vi "Create Find and Replace Array for Word.vi"(7 "Language":string, 8 "error in":errorcluster, 10 "Mathcad Output":T1, 11 "DesignRequest":T2) -> (0 "error out":errorcluster, 3 "Find-Replace":cluster{"Find":string, "Replace":string}[](array[cluster]))   [LabVIEW 2012, in "Design Server.lvlib"]
uses:
  Design Server.lvlib
  Design Request.ctl
  Variable cluster.ctl
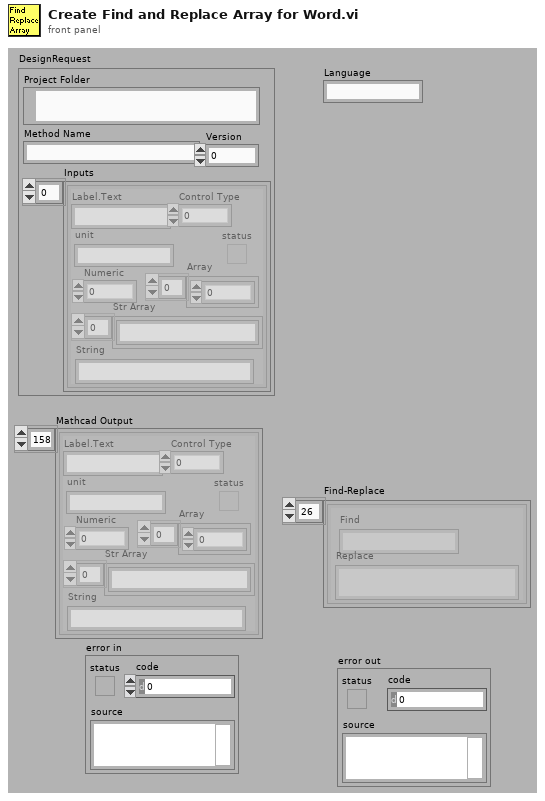
[diagram p1: front panel]
types:
  T1 = typedef "Design Server.lvlib/Variable cluster.ctl" = cluster{"Label.Text":string, "Control Type":u32, "Numeric":dbl, "Array":dbl[], "status":bool, "Str Array":string[], "String":string, "unit":string}[]
  T2 = typedef "Design Server.lvlib/Design Request.ctl" = cluster{"Project Folder":path, "Method Name":string, "Inputs":T1, "Version":i32}
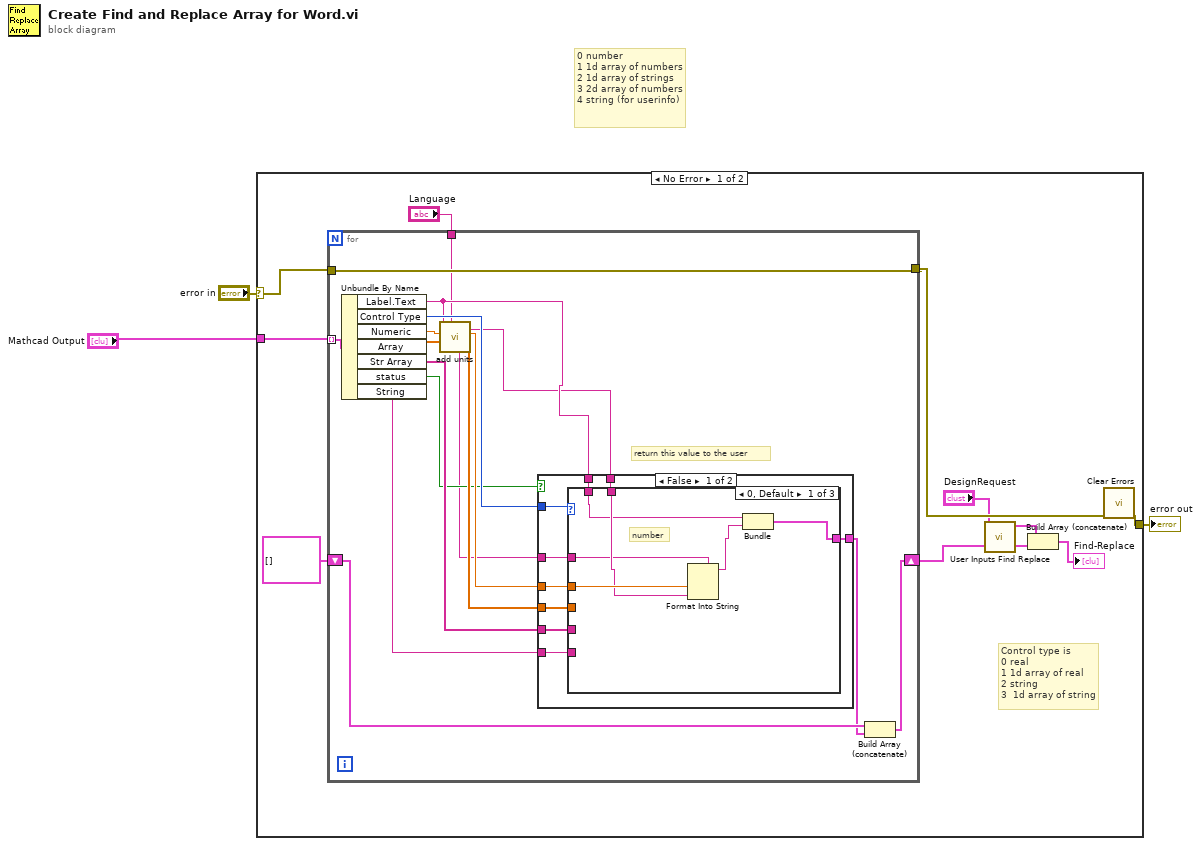
[diagram p0: block diagram]
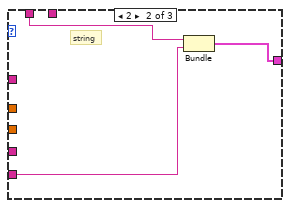
[diagram p2: hidden frame]
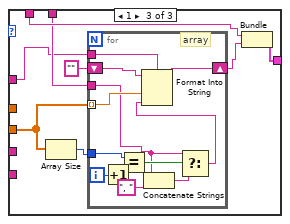
[diagram p3: hidden frame]
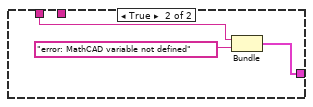
[diagram p4: hidden frame]
diagram:
  # "0\tnumber\n1\t1d array of numbers\n2\t1d array of strings\n3\t2d array of numbers\n4 string (for userinfo)"
  n1 = case shown="No Error" "error in" {
    selector: "error in" -> [w9 w72]
    tunnel: [w12 w72] -> w3
    tunnel: "Mathcad Output" -> [w11 _]
    frame No Error {
      # "Control type is\n0 real\n1 1d array of real\n2 string\n3  1d array of string"
      n2 = for {
        tunnel: w9 -> [w28]
        tunnel: [w28] -> w8
        tunnel: w11 -> [w30] mode=indexing
        shift-right: [w18] -> w13
        shift-left: cluster{"Label.Text":string, "string":string}[] [] -> [w19]
        tunnel: "Language" -> [w14]
        # "return this value to the user"
        n3 = Unbundle By Name(w30) -> ("Label.Text"=w21:string, "Control Type"=w29:u32, "Numeric"=w25:dbl, "Array"=w26:dbl[], "Str Array"=w27:string[], "status"=w22:bool, "String"=w16:string)
        n4 = call "add units.vi"("Language"=w14, "Array"=w26, "Numeric"=w25, "Label Text"=w21) -> ("Converted Array"=w24:dbl[], "Converted Numeric"=w23:dbl, "format string"=w17:string, "unit"=w20:string)  [unwired: 3 in, 1 out]
        n5 = case shown="False" w22 {
          tunnel: w29 -> [w39 _]
          tunnel: w23 -> [w38 _]
          tunnel: w24 -> [w37 _]
          tunnel: w20 -> [w36 _]
          tunnel: [w35 w70] -> w15
          tunnel: w27 -> [w34 _]
          tunnel: w21 -> [w33 w71]
          tunnel: w17 -> [w32 _]
          tunnel: w16 -> [w31 _]
          frame False {
            n6 = case shown="0, Default" w39 {
              tunnel: [w41 w47 w54] -> w35
              tunnel: w38 -> [w45 _ _]
              tunnel: w37 -> [_ _ w55]
              tunnel: w36 -> [w44 _ w51]
              tunnel: w34 -> [_ _ _]
              tunnel: w33 -> [w43 w48 w53]
              tunnel: w32 -> [w40 _ w49]
              tunnel: w31 -> [_ w46 _]
              frame 0, Default {
                # "number"
                n7 = Format Into String(format string=w40, w45, w44) -> (resulting string=w42:string)  [unwired: 2 in, 1 out]
                n8 = Bundle("Label.Text"=w43, w42) -> (w41:cluster{"Label.Text":string, string})  [unwired: 1 in]
              }
              frame 2 {
                # "string"
                n9 = Bundle("Label.Text"=w48, "String"=w46) -> (w47:cluster{"Label.Text":string, "String":string})  [unwired: 1 in]
              }
              frame 1 {
                n10 = Array Size(array=w55) -> (size(s)=w56:i32)
                n11 = for {
                  shift-right: [w68] -> w52
                  shift-left: "" -> [w62]
                  tunnel: w55 -> [w63] mode=indexing
                  tunnel: w56 -> [w65]
                  tunnel: w51 -> [w58]
                  tunnel: w49 -> [w61]
                  i -> [w67]
                  # "array"
                  n12 = Increment(x=w67) -> (x+1=w64:i32)
                  n13 = Equal?(x=w65, y=w64) -> (x = y?=w66:bool)
                  n14 = Concatenate Strings(w58, ", " ("string")) -> (w60:string)
                  n15 = Select(t=w58, s=w66, f=w60) -> (s? t:f=w57:string)
                  n16 = Format Into String(format string=w61, initial string=w62, w63, w57) -> (resulting string=w68:string)  [unwired: 1 in, 1 out]
                }
                n17 = Bundle("Label.Text"=w53, w52) -> (w54:cluster{"Label.Text":string, string})  [unwired: 1 in]
              }
            }
          }
          frame True {
            n18 = Bundle("Label.Text"=w71, "string"="error: MathCAD variable not defined") -> (w70:cluster{"Label.Text":string, "string":string})  [unwired: 1 in]
          }
        }
        n19 = Build Array (concatenate)(w19, w15) -> (w18:cluster{"Label.Text":string, "string":string}[])
      }
      n20 = call "User Inputs Find Replace.vi"("DesignRequest"="DesignRequest") -> ("Find-Replace"=w5:cluster{"Find":string, "Replace":string}[])  [unwired: 10 in]
      n21 = Build Array (concatenate)(w5, w13) -> (→"Find-Replace":cluster{"Label.Text":string, "string":string}[])
      n22 = call <vilib>:"Clear Errors.vi"("error in (no error)"=w8) -> ("error out"=w12:errorcluster)  [unwired: 6 in]
    }
    frame Error {
    }
  }
  "error out" <- w3
